vi "Coin Counter Two.vi"() -> ()   [LabVIEW 2017]
panel:
  out "?":dbl(slide) scale=0.0..100.0
  out "Money ($)":dbl
  in  "Coin":string
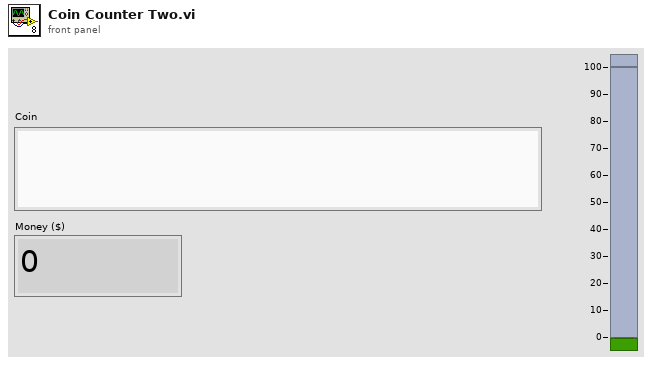
[diagram p1: front panel]
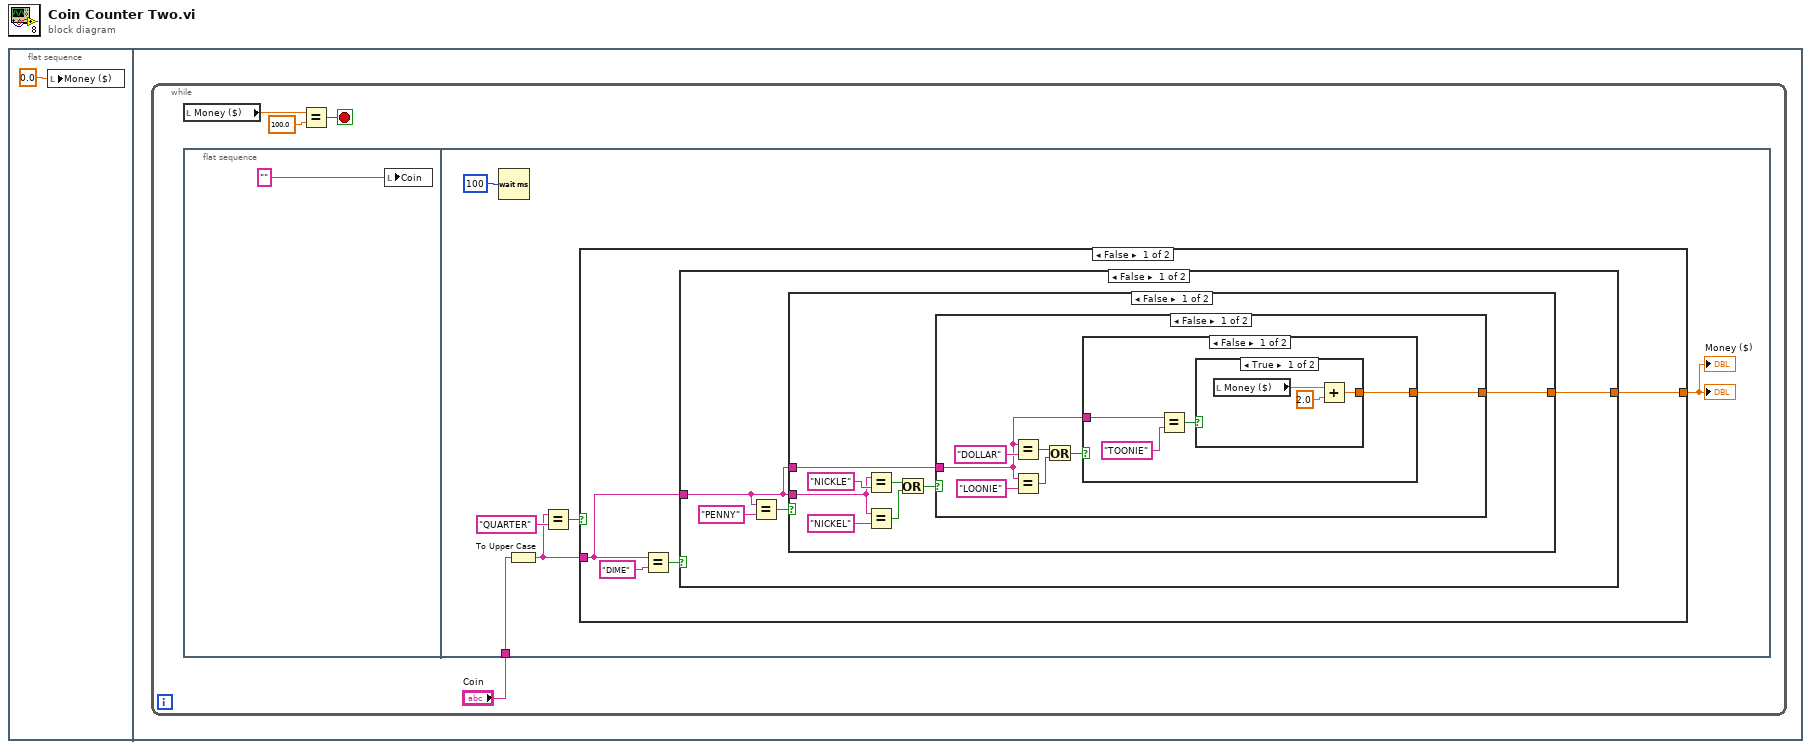
[diagram p0: block diagram]
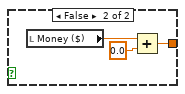
[diagram p2: hidden frame]
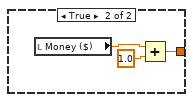
[diagram p3: hidden frame]
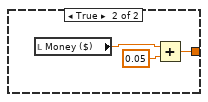
[diagram p4: hidden frame]
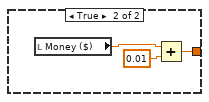
[diagram p5: hidden frame]
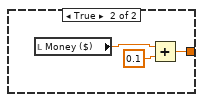
[diagram p6: hidden frame]
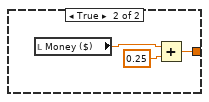
[diagram p7: hidden frame]
diagram:
  n1 = flat-sequence {
    frame #0 {
      n2 = local write "Money ($)"(0.0 ("Sum")) -> ()
    }
    frame #1 {
      n3 = while {
        stop <- w3 stop-if-true
        n4 = local read "Money ($)"() -> (w5:dbl)
        n5 = flat-sequence {
          tunnel: "Coin" -> [w7]
          frame #0 {
            n6 = local write "Coin"("") -> ()
          }
          frame #1 {
            n7 = Wait (ms)(milliseconds to wait=u32 100) -> ()  [unwired: 1 out]
            n8 = To Upper Case(1:w7) -> (0:w9:string)
            n9 = Equal?(x=w9, y="QUARTER") -> (x = y?=w11:bool)
            n10 = case shown="False" w11 {
              tunnel: [w15 w58] -> w8
              tunnel: w9 -> [w13 _]
              frame False {
                n11 = Equal?(x=w13, y="DIME") -> (x = y?=w14:bool)
                n12 = case shown="False" w14 {
                  tunnel: [w18 w55] -> w15
                  tunnel: w13 -> [w17 _]
                  frame False {
                    n13 = Equal?(x=w17, y="PENNY") -> (x = y?=w19:bool)
                    n14 = case shown="False" w19 {
                      tunnel: [w22 w52] -> w18
                      tunnel: w17 -> [w26 _]
                      tunnel: w17 -> [w21 _]
                      frame False {
                        n15 = Equal?(x=w26, y="NICKLE") -> (x = y?=w25:bool)
                        n16 = Equal?(x=w26, y="NICKEL") -> (x = y?=w24:bool)
                        n17 = Or(x=w25, y=w24) -> (x .or. y?=w23:bool)
                        n18 = case shown="False" w23 {
                          tunnel: [w30 w49] -> w22
                          tunnel: w21 -> [w29 _]
                          frame False {
                            n19 = Equal?(x=w29, y="DOLLAR") -> (x = y?=w34:bool)
                            n20 = Equal?(x=w29, y="LOONIE") -> (x = y?=w35:bool)
                            n21 = Or(x=w34, y=w35) -> (x .or. y?=w31:bool)
                            n22 = case shown="False" w31 {
                              tunnel: [w36 w46] -> w30
                              tunnel: w29 -> [w39 _]
                              frame False {
                                n23 = Equal?(x=w39, y="TOONIE") -> (x = y?=w37:bool)
                                n24 = case shown="True" w37 {
                                tunnel: [w40 w43] -> w36
                                frame True {
                                n25 = local read "Money ($)"() -> (w42:dbl)
                                n26 = Add(x=w42, y=2.0) -> (x+y=w40:dbl)
                                }
                                frame False {
                                n27 = local read "Money ($)"() -> (w45:dbl)
                                n28 = Add(x=w45, y=0.0) -> (x+y=w43:dbl)
                                }
                                }
                              }
                              frame True {
                                n29 = local read "Money ($)"() -> (w48:dbl)
                                n30 = Add(x=w48, y=1.0) -> (x+y=w46:dbl)
                              }
                            }
                          }
                          frame True {
                            n31 = local read "Money ($)"() -> (w51:dbl)
                            n32 = Add(x=w51, y=0.05) -> (x+y=w49:dbl)
                          }
                        }
                      }
                      frame True {
                        n33 = local read "Money ($)"() -> (w54:dbl)
                        n34 = Add(x=w54, y=0.01) -> (x+y=w52:dbl)
                      }
                    }
                  }
                  frame True {
                    n35 = local read "Money ($)"() -> (w57:dbl)
                    n36 = Add(x=w57, y=0.1) -> (x+y=w55:dbl)
                  }
                }
              }
              frame True {
                n37 = local read "Money ($)"() -> (w60:dbl)
                n38 = Add(x=w60, y=0.25) -> (x+y=w58:dbl)
              }
            }
            "?" <- w8
            "Money ($)" <- w8
          }
        }
        n39 = Equal?(x=w5, y=100.0) -> (x = y?=w3:bool)
      }
    }
  }
